vi "Build Caraya to PPL.vi"() -> ()   [LabVIEW 2020]
uses:
  <vilib>/AppBuilder/AB_API_Simple/Build (path).vi
  Caraya.lvlib
  <vilib>/AppBuilder/AB_API_Simple/NI_App_Builder_API.lvlib
panel:
  in  "Build Caraya PPL":bool
  in  "Destination Folder":path
  in  "Caraya PPL filename":string="Caraya"
  # "CARAYA PPL Builder\n\nFill in the destination folder and PPL filename."
  # ".lvlibp"
  # "Note: \nIt is recommended that you do not change the PPL filename."
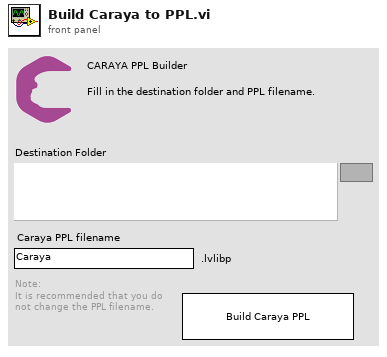
[diagram p1: front panel]
types:
  T1 = enum32{"invalid app kind", "Development System", "Run Time System", "Student Edition", "Embedded LabVIEW", "Evaluation", "Custom"}
  T2 = enum8{"Enabled", "Disabled", "Disabled and Grayed Out"}
  T3 = enum32{"Invalid", "Standard", "Closed", "Hidden", "Minimized", "Maximized"}
  T4 = cluster{"Core":cluster{"Current VI Reference":refnum<vi>, "Close Panel on Exit?":bool}, "PPL Filename":string, "Path":path, "Menu Launch AppRef":refnum<vi>, "Projects[]":refnum<vi>[]}
  T5 = cluster{"Current VI Reference":refnum<vi>, "Close Panel on Exit?":bool}
  T6 = typedef "Caraya.lvlib/Caraya Library Info.ctl" = cluster{"Version String":string, "Name":string, "Copyright":string, "License":string}
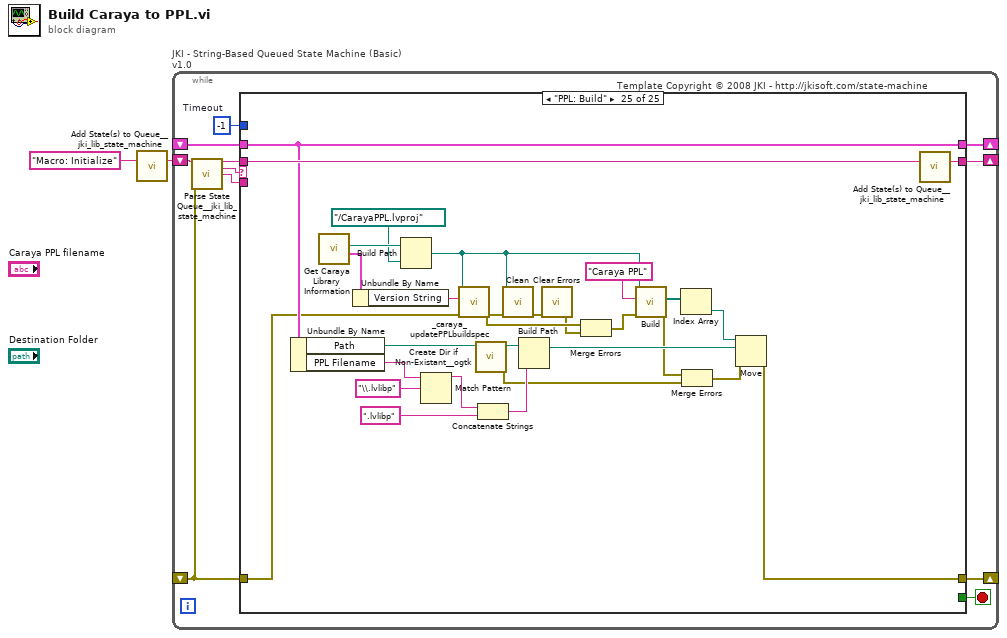
[diagram p0: block diagram]
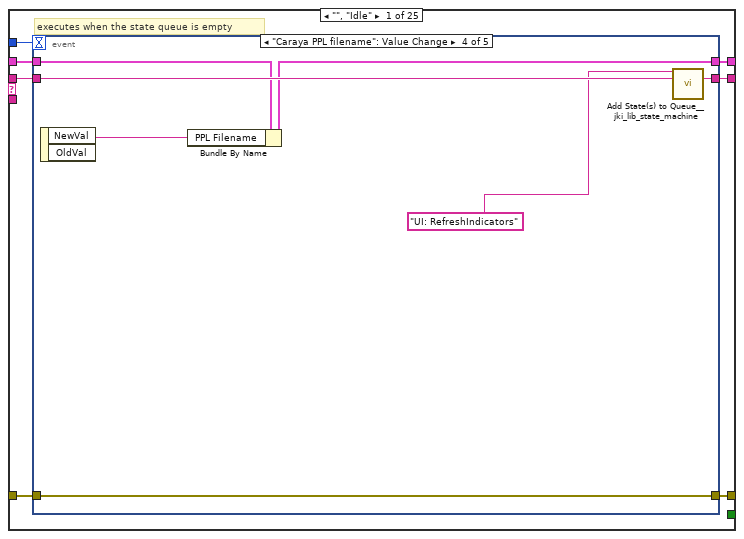
[diagram p2: hidden frame]
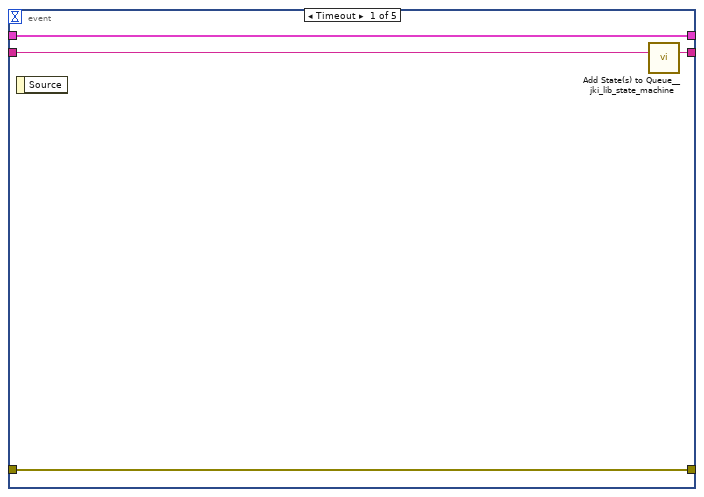
[diagram p3: hidden frame]
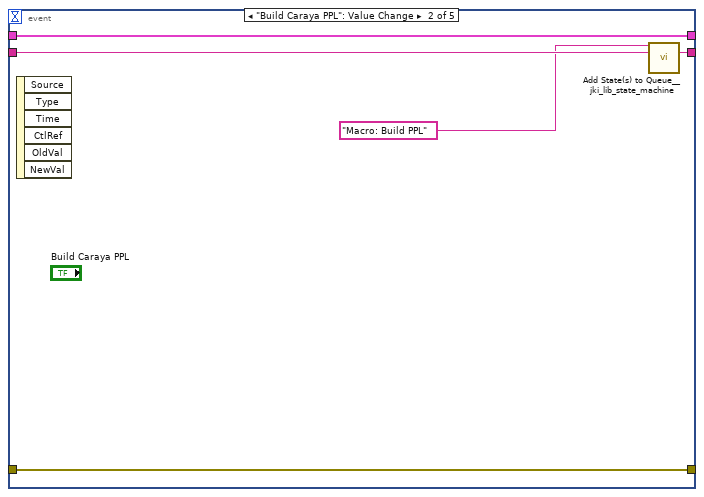
[diagram p4: hidden frame]
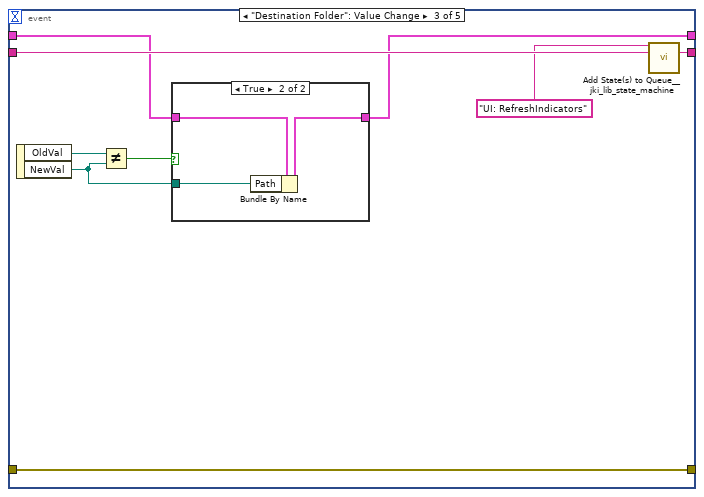
[diagram p5: hidden frame]
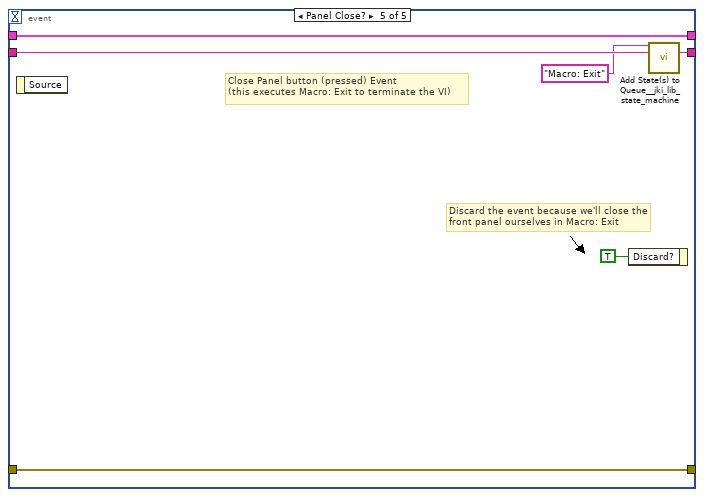
[diagram p7: hidden frame]
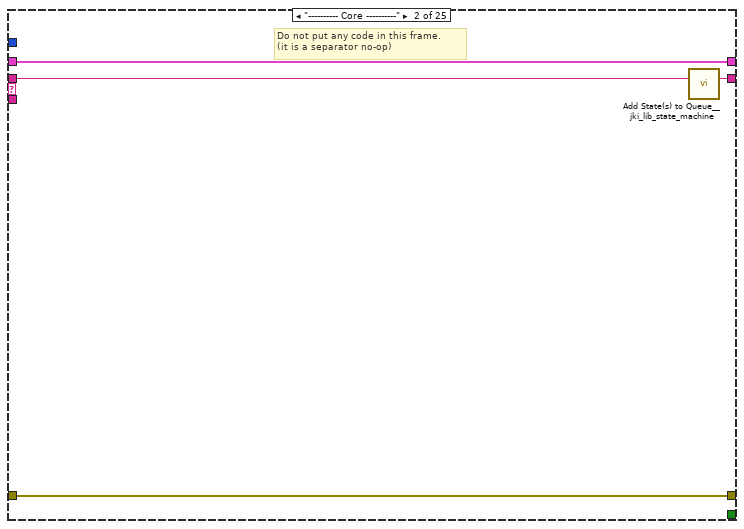
[diagram p8: hidden frame]
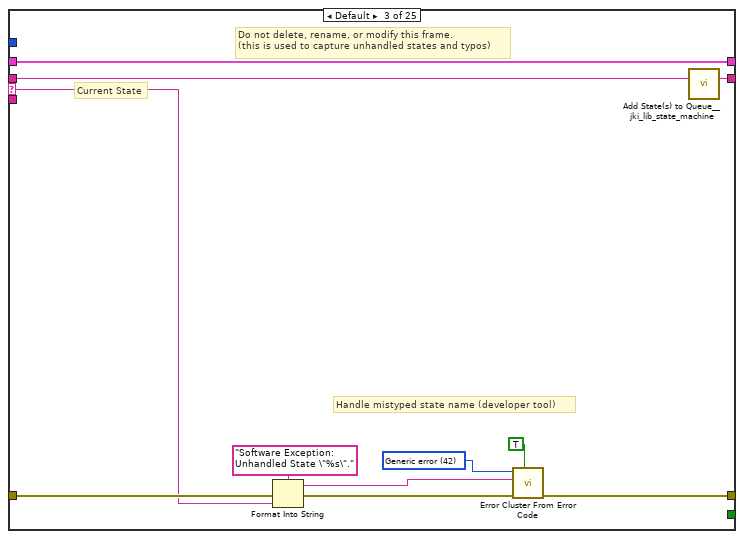
[diagram p9: hidden frame]
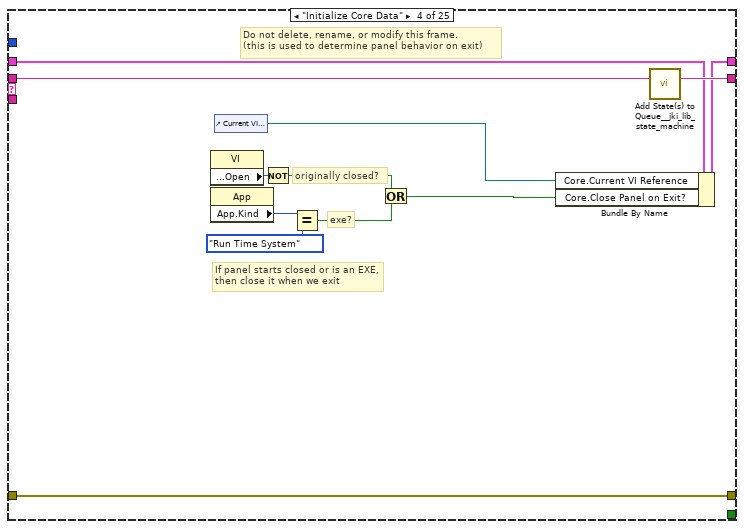
[diagram p10: hidden frame]
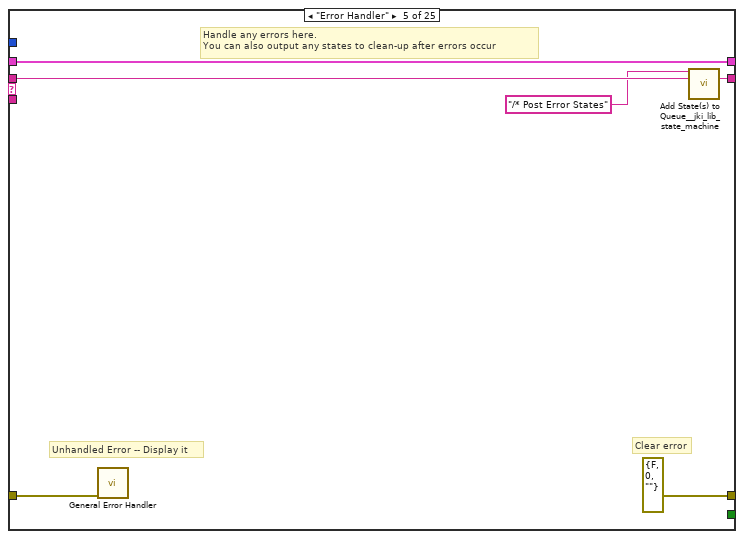
[diagram p11: hidden frame]
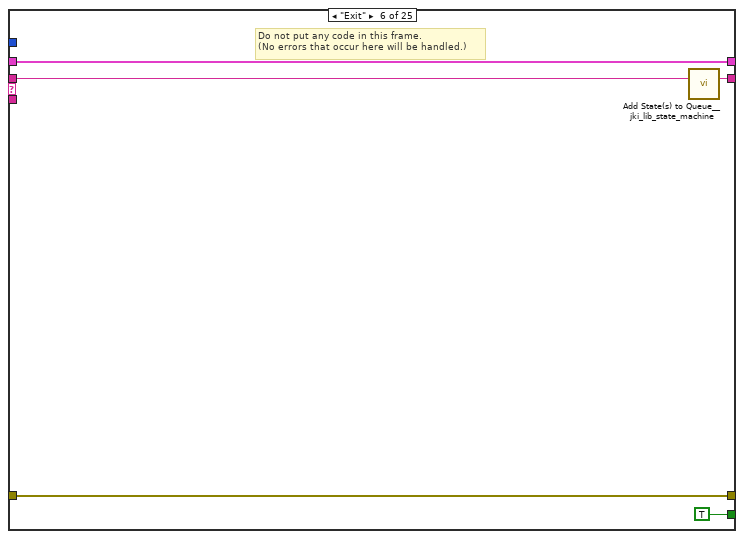
[diagram p12: hidden frame]
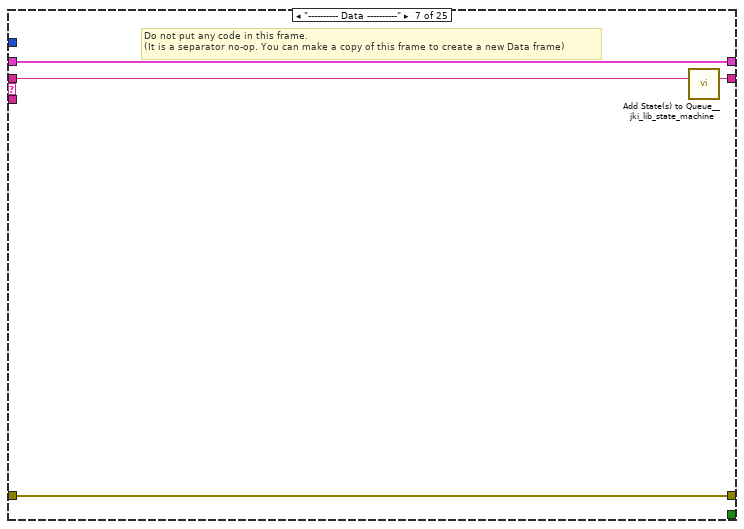
[diagram p13: hidden frame]
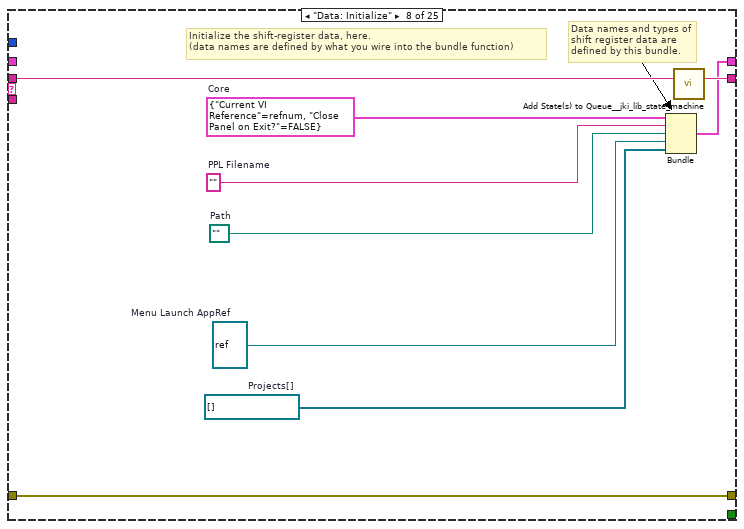
[diagram p14: hidden frame]
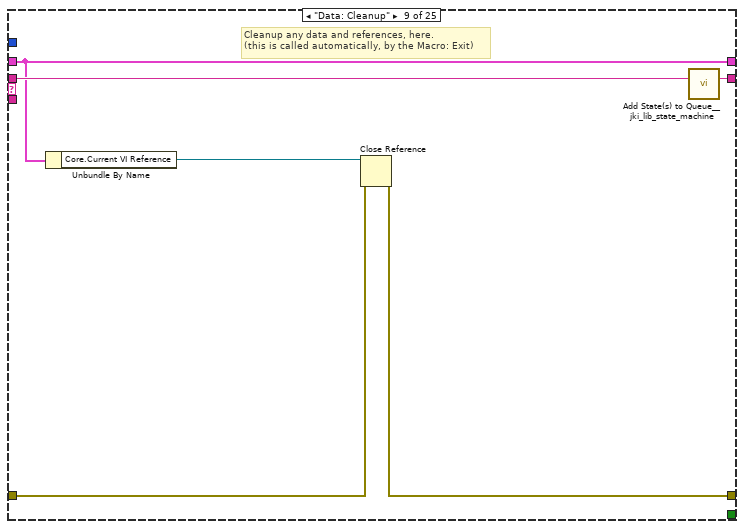
[diagram p15: hidden frame]
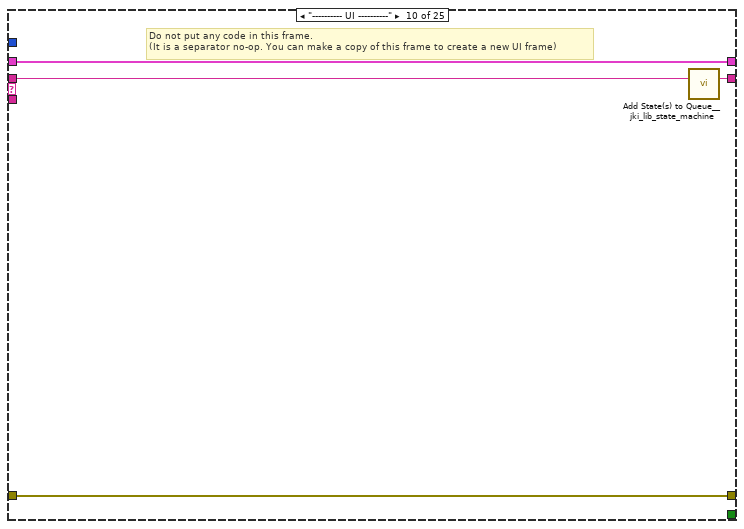
[diagram p16: hidden frame]
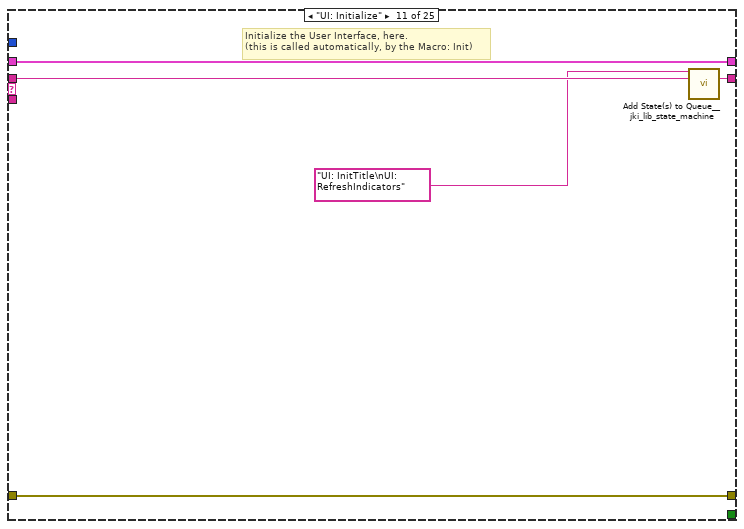
[diagram p17: hidden frame]
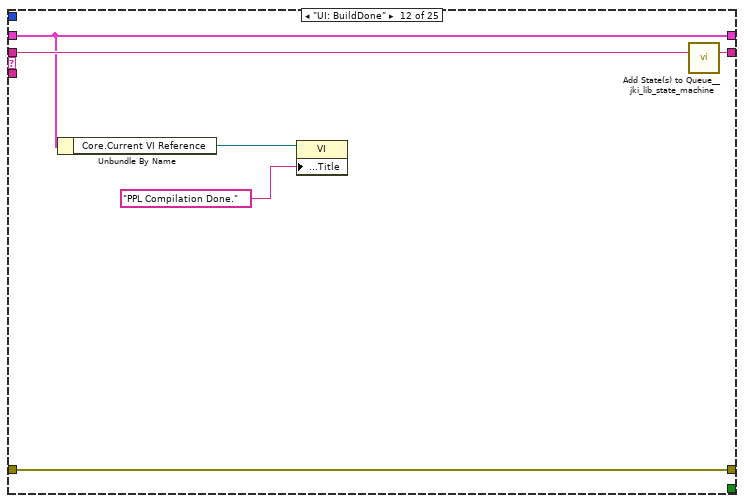
[diagram p18: hidden frame]
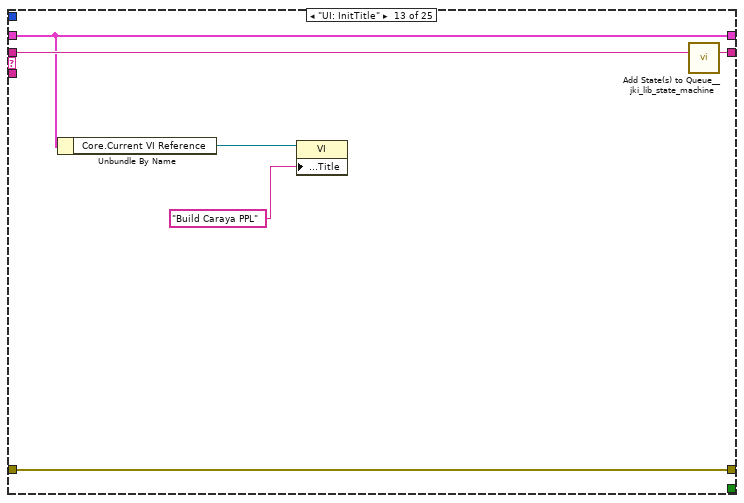
[diagram p19: hidden frame]
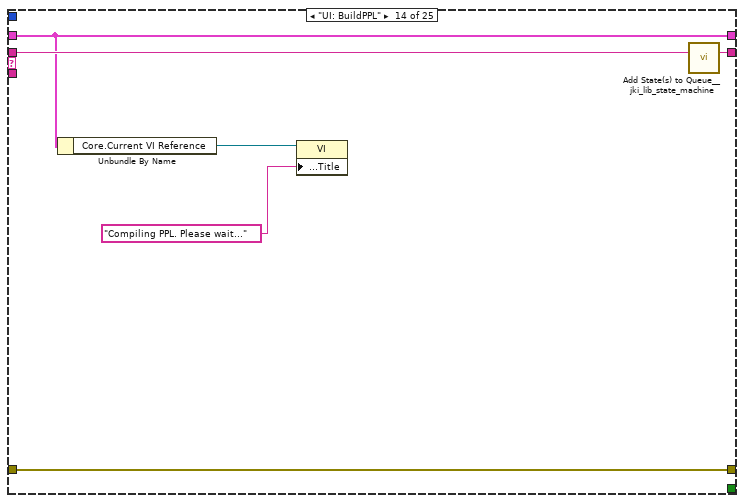
[diagram p20: hidden frame]
diagram:
  n1 = call <vilib>:"Add State(s) to Queue__jki_lib_state_machine.vi"("State(s) in (\"\")"="Macro: Initialize") -> ("States Out"=w2:string)  [unwired: 14 in]
  n2 = while "JKI - String-Based Queued State Machine (Basic) v1.0" {
    shift-right: [w6] -> _
    shift-left: _ -> [w5]
    shift-right: [w9] -> _
    shift-left: _ -> [w3]
    shift-right: [w8] -> _
    shift-left: w2 -> [w10]
    stop <- w7 stop-if-true
    w4 = -1  # Timeout
    # "Template Copyright © 2008 JKI - http://jkisoft.com/state-machine"
    n3 = call <vilib>:"Parse State Queue__jki_lib_state_machine.vi"("State Queue"=w10, "Error In (no error)"=w3) -> ("Remaining States"=w12:string, "Current State"=w13:string, "Arguments"=w11:string)  [unwired: 11 in]
    n4 = case shown="\"PPL: Build\"" w13 {
      selector: w13 -> [_ _ w60 _ _ _ _ _ _ _ _ _ _ _ _ _ _ _ _ _ _ _ _ _ _]
      tunnel: w12 -> [w20 w59 w64 w82 w88 w93 w97 w106 w112 w116 w121 w127 w133 w139 w152 w158 w169 w195 w200 w205 w212 w216 w222 w232 w262]
      tunnel: w11 -> [_ _ _ _ _ _ _ _ _ _ _ _ _ _ _ w153 w163 _ _ _ _ _ _ _ _]
      tunnel: w5 -> [w18 w56 w62 w73 w85 w91 w94 _ w107 w113 w118 w124 w130 w136 w140 w156 w165 w192 w197 w202 w209 w213 w218 w223 w260]
      tunnel: [w17 w57 w66 w79 errorcluster {"status"=FALSE, "code"=0, "source"=""} ("error out") w90 w95 w103 w108 w114 w119 w125 w131 w137 w150 w154 w166 w193 w198 w203 w210 w214 w220 w230 w241] -> w9
      tunnel: w3 -> [w16 w57 w65 w79 w84 w90 w95 w103 w109 w114 w119 w125 w131 w137 w150 w155 w167 w193 w198 w203 w210 w214 w220 w230 w247]
      tunnel: [w19 w58 w63 w81 w87 w92 w96 w105 w111 w115 w120 w126 w132 w138 w151 w157 w168 w194 w199 w204 w211 w215 w221 w231 w261] -> w8
      tunnel: [_ _ _ _ _ TRUE _ _ _ _ _ _ _ _ _ _ _ _ _ _ _ _ _ _ _] -> w7
      tunnel: [w15 w56 w62 w80 w85 w91 w94 w104 w107 w113 w118 w124 w130 w136 w140 w156 w165 w192 w197 w202 w209 w213 w217 w229 w260] -> w6
      tunnel: w4 -> [w14 _ _ _ _ _ _ _ _ _ _ _ _ _ _ _ _ _ _ _ _ _ _ _ _]
      frame "", "Idle" {
        # "executes when the state queue is empty"
        n5 = event shown="[3] \"Caraya PPL filename\": Value Change" {
          selector: _ -> [_ _ _ _ _]
          dyn-events: _ -> [_ _ _ _ _]
          timeout: w14 -> [_ _ _ _ _]
          tunnel: w20 -> [w24 w29 w38 w49 w55]
          tunnel: [w23 w28 w37 w48 w54] -> w19
          tunnel: w18 -> [w21 w26 w34 w46 w52]
          tunnel: [w22 w27 w36 w47 w53] -> w17
          tunnel: w16 -> [w22 w27 w36 w47 w53]
          tunnel: [w21 w26 w31 w45 w52] -> w15
          event Timeout {
            n6 = event-data() -> ()  [unwired: 1 in, 1 out]
            n7 = call <vilib>:"Add State(s) to Queue__jki_lib_state_machine.vi"("State(s) in (\"\")"=w24) -> ("States Out"=w23:string)  [unwired: 14 in]
          }
          event "Build Caraya PPL": Value Change {
            n8 = event-data() -> ()  [unwired: 1 in, 6 out]
            n9 = call <vilib>:"Add State(s) to Queue__jki_lib_state_machine.vi"("State(s) in Front (\"\")"="Macro: Build PPL", "State(s) in (\"\")"=w29) -> ("States Out"=w28:string)  [unwired: 13 in]
          }
          event "Destination Folder": Value Change {
            n10 = event-data() -> ("OldVal"=w35:path, "NewVal"=w32:path)  [unwired: 1 in]
            n11 = Not Equal?(x=w35, y=w32) -> (x != y?=w33:bool)
            n12 = case shown="True" w33 {
              tunnel: [w39 w42] -> w31
              tunnel: w34 -> [w39 w41]
              tunnel: w32 -> [_ w40]
              frame False {
              }
              frame True {
                n13 = Bundle By Name(cluster=w41, "Path"=w40) -> (w42:T4)
              }
            }
            n14 = call <vilib>:"Add State(s) to Queue__jki_lib_state_machine.vi"("State(s) in Front (\"\")"="UI: RefreshIndicators", "State(s) in (\"\")"=w38) -> ("States Out"=w37:string)  [unwired: 13 in]
          }
          event "Caraya PPL filename": Value Change {
            n15 = event-data() -> ("NewVal"=w44:string)  [unwired: 1 in, 1 out]
            n16 = Bundle By Name(cluster=w46, "PPL Filename"=w44) -> (w45:T4)
            n17 = call <vilib>:"Add State(s) to Queue__jki_lib_state_machine.vi"("State(s) in Front (\"\")"="UI: RefreshIndicators", "State(s) in (\"\")"=w49) -> ("States Out"=w48:string)  [unwired: 13 in]
          }
          event Panel Close? {
            # "Discard the event because we'll close the front panel ourselves in Macro: Exit"
            # "Close Panel button (pressed) Event\n(this executes Macro: Exit to terminate the VI)"
            n18 = event-data() -> ()  [unwired: 1 in, 1 out]
            n19 = event-data("Discard?"=TRUE) -> ()  [unwired: 1 in, 1 out]
            n20 = call <vilib>:"Add State(s) to Queue__jki_lib_state_machine.vi"("State(s) in Front (\"\")"="Macro: Exit", "State(s) in (\"\")"=w55) -> ("States Out"=w54:string)  [unwired: 13 in]
          }
        }
      }
      frame "---------- Core ----------" {
        # "Do not put any code in this frame.\n(it is a separator no-op)"
        n21 = call <vilib>:"Add State(s) to Queue__jki_lib_state_machine.vi"("State(s) in (\"\")"=w59) -> ("States Out"=w58:string)  [unwired: 14 in]
      }
      frame Default {
        w69 = 42 items=["No error", "Argument error", "Memory is full", "Out of zone", "End of file", "File already open", "Generic file I/O error", "File not found", "File permission error", "Disk is full", "Duplicate path", "Too many files open", "System feature not enabled", "Resource file not found", "Cannot add resource", "Resource not found", "Image not found", "Image memory error", "Pen does not exist", "Config type invalid", "Config token not found", "Config parse error", "Config memory error", "Bad external code format", "Bad external code offset", "External code not present", "Null window", "Destroy window error", "Null menu", "Print aborted", "Bad print record", "Print driver error", "Windows error during printing", "Memory error during printing", "Print dialog error", "Generic print error", "Invalid device refnum", "Device not found", "Device parameter error", "Device unit error", "Cannot open device", "Device call aborted", "Generic error", "Cancelled by user", "Object ID too low", "Object ID too high", "Object not in heap", "Unknown heap", "Unknown object (invalid DefProc)", "Unknown object (DefProc not in table)", "Message out of range", "Invalid (null) method", "Unknown message", "Manager call not supported", "Bad address", "Network operation in progress", "Network operation timed out", "Connection is busy", "Network attribute not supported", "Network error", "Address in use", "System out of memory", "Connection aborted", "Connection refused", "Not connected", "Already connected", "Connection closed", "Initialization error (interapplication manager)", "Bad occurrence", "Wait on unbound occurrence handler", "Occurrence queue overflow", "Datalog type conflict", "Unused", "Unrecognized type (interapplication manager)", "Memory corrupt", "Failed to make temporary DLL", "Old CIN version", "Drag socket not found", "Failed to load drop-object", "Failed to register OLE object", "Failed to release OLE object", "Format specifier type mismatch", "Unknown format specifier", "Too few format specifiers", "Too many format specifiers", "Scan failed", "Newer CIN version", "Error converting to variant", "Runtime menu error", "Password tampered", "Variant attribute not found", "Incompatible variant data type", "Event data is not available", "Event Store is not present", "Occurrence is not found", "Event Queue is not created", "Event info is not available", "Refnum passed is NULL", "Error retrieving Class GUID", "Error retrieving CoClass GUID", "Error retrieving TypeLib GUID.", "Bad built application magic bytes.", "Specific driver is different from the specific driver associated with the Logical Name.", "There is no session opened to the class driver.", "Max Error", "MAX - Error with config objects", "MAX - Error loading configuration", "MAX - Group not supported"]
        # "Current State"
        # "Do not delete, rename, or modify this frame.\n(this is used to capture unhandled states and typos)"
        # "Handle mistyped state name (developer tool)"
        n22 = Format Into String(format string="Software Exception: Unhandled State \"%s\"." ("message"), error in=w65, w60) -> (resulting string=w68:string, error out=w67:errorcluster)  [unwired: 1 in]
        n23 = call <vilib>:"Error Cluster From Error Code.vi"("show call chain? (False)"=TRUE, "error in (no error)"=w67, "error message (\"\")"=w68, "error code (0)"=w69) -> ("error out"=w66:errorcluster)  [unwired: 5 in]
        n24 = call <vilib>:"Add State(s) to Queue__jki_lib_state_machine.vi"("State(s) in (\"\")"=w64) -> ("States Out"=w63:string)  [unwired: 14 in]
      }
      frame "Initialize Core Data" {
        # "Do not delete, rename, or modify this frame.\n(this is used to determine panel behavior on exit)"
        # "originally closed?"
        # "exe?"
        # "If panel starts closed or is an EXE, then close it when we exit"
        n25 = property class="VI"() -> ("Front Panel.Open"=w78:bool)  [unwired: 2 in, 2 out]
        n26 = property class="App"() -> ("App.Kind"=w77:T1)  [unwired: 2 in, 2 out]
        n27 = control-ref of="Current VI Reference"() -> (w71:refnum<vi>)
        n28 = Not(x=w78) -> (.not. x?=w75:bool)
        n29 = Equal?(x=w77, y=T1."Run Time System" ("Application:Kind")) -> (x = y?=w74:bool)
        n30 = Or(x=w75, y=w74) -> (x .or. y?=w72:bool)
        n31 = Bundle By Name(cluster=w73, "Core.Current VI Reference"=w71, "Core.Close Panel on Exit?"=w72) -> (w80:T4)
        n32 = call <vilib>:"Add State(s) to Queue__jki_lib_state_machine.vi"("State(s) in (\"\")"=w82) -> ("States Out"=w81:string)  [unwired: 14 in]
      }
      frame "Error Handler" {
        # "Unhandled Error -- Display it"
        # "Handle any errors here.\nYou can also output any states to clean-up after errors occur"
        # "Clear error"
        n33 = call <vilib>:"General Error Handler.vi"("error in (no error)"=w84) -> ()  [unwired: 10 in, 5 out]
        n34 = call <vilib>:"Add State(s) to Queue__jki_lib_state_machine.vi"("State(s) in Front (\"\")"="/* Post Error States", "State(s) in (\"\")"=w88) -> ("States Out"=w87:string)  [unwired: 13 in]
      }
      frame "Exit" {
        # "Do not put any code in this frame.\n(No errors that occur here will be handled.)"
        n35 = call <vilib>:"Add State(s) to Queue__jki_lib_state_machine.vi"("State(s) in (\"\")"=w93) -> ("States Out"=w92:string)  [unwired: 14 in]
      }
      frame "---------- Data ----------" {
        # "Do not put any code in this frame.\n(It is a separator no-op. You can make a copy of this frame to create a new Data frame)"
        n36 = call <vilib>:"Add State(s) to Queue__jki_lib_state_machine.vi"("State(s) in (\"\")"=w97) -> ("States Out"=w96:string)  [unwired: 14 in]
      }
      frame "Data: Initialize" {
        w98 = refnum<vi>[] []  # Projects[]
        w99 = refnum<vi> refnum  # Menu Launch AppRef
        w100 = path ""  # Path
        w101 = T5 {"Current VI Reference"=refnum, "Close Panel on Exit?"=FALSE}  # Core
        w102 = ""  # PPL Filename
        # "Data names and types of shift register data are defined by this bundle."
        # "Initialize the shift-register data, here.\n(data names are defined by what you wire into the bundle function)"
        n37 = Bundle("Core"=w101, "PPL Filename"=w102, "Path"=w100, "Menu Launch AppRef"=w99, "Projects[]"=w98) -> (w104:T4)  [unwired: 1 in]
        n38 = call <vilib>:"Add State(s) to Queue__jki_lib_state_machine.vi"("State(s) in (\"\")"=w106) -> ("States Out"=w105:string)  [unwired: 14 in]
      }
      frame "Data: Cleanup" {
        # "Cleanup any data and references, here.\n(this is called automatically, by the Macro: Exit)"
        n39 = Unbundle By Name(w107) -> ("Core.Current VI Reference"=w110:refnum<vi>)
        n40 = Close Reference(reference=w110, error in (no error)=w109) -> (error out=w108:errorcluster)
        n41 = call <vilib>:"Add State(s) to Queue__jki_lib_state_machine.vi"("State(s) in (\"\")"=w112) -> ("States Out"=w111:string)  [unwired: 14 in]
      }
      frame "---------- UI ----------" {
        # "Do not put any code in this frame.\n(It is a separator no-op. You can make a copy of this frame to create a new UI frame)"
        n42 = call <vilib>:"Add State(s) to Queue__jki_lib_state_machine.vi"("State(s) in (\"\")"=w116) -> ("States Out"=w115:string)  [unwired: 14 in]
      }
      frame "UI: Initialize" {
        # "Initialize the User Interface, here.\n(this is called automatically, by the Macro: Init)"
        n43 = call <vilib>:"Add State(s) to Queue__jki_lib_state_machine.vi"("State(s) in Front (\"\")"="UI: InitTitle\nUI: RefreshIndicators" ("Text.Text"), "State(s) in (\"\")"=w121) -> ("States Out"=w120:string)  [unwired: 13 in]
      }
      frame "UI: BuildDone" {
        n44 = Unbundle By Name(w124) -> ("Core.Current VI Reference"=w123:refnum<vi>)
        n45 = property class="VI"(reference=w123, "Front Panel.Title"="PPL Compilation Done." ("Front Panel Window:Title")) -> ()  [unwired: 1 in, 2 out]
        n46 = call <vilib>:"Add State(s) to Queue__jki_lib_state_machine.vi"("State(s) in (\"\")"=w127) -> ("States Out"=w126:string)  [unwired: 14 in]
      }
      frame "UI: InitTitle" {
        n47 = Unbundle By Name(w130) -> ("Core.Current VI Reference"=w129:refnum<vi>)
        n48 = property class="VI"(reference=w129, "Front Panel.Title"="Build Caraya PPL" ("Front Panel Window:Title")) -> ()  [unwired: 1 in, 2 out]
        n49 = call <vilib>:"Add State(s) to Queue__jki_lib_state_machine.vi"("State(s) in (\"\")"=w133) -> ("States Out"=w132:string)  [unwired: 14 in]
      }
      frame "UI: BuildPPL" {
        n50 = Unbundle By Name(w136) -> ("Core.Current VI Reference"=w135:refnum<vi>)
        n51 = property class="VI"(reference=w135, "Front Panel.Title"="Compiling PPL. Please wait..." ("Front Panel Window:Title")) -> ()  [unwired: 1 in, 2 out]
        n52 = call <vilib>:"Add State(s) to Queue__jki_lib_state_machine.vi"("State(s) in (\"\")"=w139) -> ("States Out"=w138:string)  [unwired: 14 in]
      }
      frame "UI: RefreshIndicators" {
        n53 = Unbundle By Name(w140) -> ("PPL Filename"=w141:string, "Path"=w142:path)
        n54 = Empty String/Path?(string/path=w141) -> (empty?=w149:bool)
        n55 = Not A Number/Path/Refnum?(number/path/refnum=w142) -> (NaN/Path/Refnum?=w148:bool)
        n56 = Empty String/Path?(string/path=w142) -> (empty?=w147:bool)
        n57 = local write "Caraya PPL filename"(w141) -> ()
        n58 = local write "Destination Folder"(w142) -> ()
        n59 = Compound Arithmetic op=OR(w149, w148, w147) -> (w145:bool)
        n60 = Select(t=T2."Disabled and Grayed Out" ("Disabled"), s=w145, f=T2."Enabled" ("Disabled")) -> (s? t:f=w143:T2)
        n61 = property on="Build Caraya PPL" class="Bool"("DisabledEnum"=w143) -> ()  [unwired: 2 in, 2 out]
        n62 = call <vilib>:"Add State(s) to Queue__jki_lib_state_machine.vi"("State(s) in (\"\")"=w152) -> ("States Out"=w151:string)  [unwired: 14 in]
      }
      frame "UI: Cursor Set" {
        # "Argument"
        # "Set and Unset Cursor Busy.\n(Usage: \"UI: Cursor Set >> Busy|Idle\")"
        n63 = case shown="\"Idle\", Default" w153 {
          tunnel: w155 -> [w160 w162]
          tunnel: [w159 w161] -> w154
          frame "Idle", Default {
            n64 = call <vilib>:"Unset Busy.vi"("error in (no error)"=w160) -> ("error out"=w159:errorcluster)  [unwired: 10 in]
          }
          frame "Busy" {
            n65 = call <vilib>:"Set Busy.vi"("error in (no error)"=w162) -> ("error out"=w161:errorcluster)  [unwired: 9 in, 1 out]
          }
        }
        n66 = call <vilib>:"Add State(s) to Queue__jki_lib_state_machine.vi"("State(s) in (\"\")"=w158) -> ("States Out"=w157:string)  [unwired: 14 in]
      }
      frame "UI: Front Panel State" {
        # "Argument"
        # "Set Front Panel Open or Closed\n(Usage: \"UI: Front Panel State >> Open|Close\")"
        n67 = Unbundle By Name(w165) -> ("Core.Current VI Reference"=w164:refnum<vi>)
        n68 = case shown="\"Open\", Default" w163 {
          tunnel: w167 -> [w173 w186]
          tunnel: [w175 w187] -> w166
          tunnel: w164 -> [w174 w184]
          frame "Open", Default {
            n69 = property class="VI"(reference=w174, error in=w173) -> (reference out=w171:refnum<vi>, error out=w172:errorcluster, "Front Panel.Open"=w170:bool)
            n70 = case shown="False" w170 {
              tunnel: [w178 w181] -> w175
              tunnel: w172 -> [w177 w181]
              tunnel: w171 -> [w176 _]
              frame False {
                n71 = invoke class="VI" method="FP.Open"(reference=w176, error in=w177, "Activate"=TRUE, "State"=T3."Standard") -> (error out=w178:errorcluster)  [unwired: 1 in, 4 out]
              }
              frame True {
              }
            }
          }
          frame "Close" {
            n72 = property class="VI"(reference=w184, error in=w186) -> (reference out=w183:refnum<vi>, error out=w185:errorcluster, "Front Panel.Open"=w182:bool)
            n73 = case shown="True" w182 {
              tunnel: [w188 w191] -> w187
              tunnel: w185 -> [w188 w190]
              tunnel: w183 -> [_ w189]
              frame False {
              }
              frame True {
                n74 = invoke class="VI" method="FP.Close"(reference=w189, error in=w190) -> (error out=w191:errorcluster)  [unwired: 1 in, 2 out]
              }
            }
          }
        }
        n75 = call <vilib>:"Add State(s) to Queue__jki_lib_state_machine.vi"("State(s) in (\"\")"=w169) -> ("States Out"=w168:string)  [unwired: 14 in]
      }
      frame "---------- Macro ----------" {
        # "Do not put any code in this frame.\n(It is a separator no-op. You can make a copy of this frame to create a new Macro frame)"
        n76 = call <vilib>:"Add State(s) to Queue__jki_lib_state_machine.vi"("State(s) in (\"\")"=w195) -> ("States Out"=w194:string)  [unwired: 14 in]
      }
      frame "Macro: Initialize" {
        w196 = "Data: Initialize\nInitialize Core Data\nPPL: Initialize Filename\nPPL: Initialize Path\nUI: Initialize\nUI: Front Panel State >> Open"  # Data: Initialize Initialize Core Data PPL: Initialize Filename PPL: Initialize Path UI: Initialize UI: Front Panel State >> Open
        # "Initialization Macro\n(This is called once, when the VI starts)"
        n77 = call <vilib>:"Add State(s) to Queue__jki_lib_state_machine.vi"("State(s) in Front (\"\")"=w196, "State(s) in (\"\")"=w200) -> ("States Out"=w199:string)  [unwired: 13 in]
      }
      frame "Macro: Build PPL" {
        n78 = call <vilib>:"Add State(s) to Queue__jki_lib_state_machine.vi"("State(s) in Front (\"\")"="UI: BuildPPL\nPPL: Build\nUI: BuildDone", "State(s) in (\"\")"=w205) -> ("States Out"=w204:string)  [unwired: 13 in]
      }
      frame "Macro: Exit" {
        # "Exit Macro\n(This is called once, when the VI exits)"
        n79 = call <vilib>:"Add State(s) to Queue__jki_lib_state_machine.vi"("State(s) in Front (\"\")"="UI: Front Panel State >> Close", "State(s) at Back (\"\")"="Data: Cleanup\nExit") -> ("States Out"=w207:string)  [unwired: 13 in]
        n80 = call <vilib>:"Add State(s) to Queue__jki_lib_state_machine.vi"("State(s) in Front (\"\")"=w207, "State(s) in (\"\")"=w212) -> ("States Out"=w211:string)  [unwired: 13 in]
      }
      frame "---------- PPL ----------" {
        n81 = call <vilib>:"Add State(s) to Queue__jki_lib_state_machine.vi"("State(s) in (\"\")"=w216) -> ("States Out"=w215:string)  [unwired: 14 in]
      }
      frame "PPL: Initialize Filename" {
        n82 = Unbundle By Name(w218) -> ()  [unwired: 1 out]
        n83 = Bundle By Name(cluster=w218, "PPL Filename"="Caraya") -> (w217:T4)
        n84 = call <vilib>:"Add State(s) to Queue__jki_lib_state_machine.vi"("State(s) in (\"\")"=w222) -> ("States Out"=w221:string)  [unwired: 14 in]
      }
      frame "PPL: Initialize Path" {
        n85 = property on="Destination Folder" class="Path"() -> ("Value"=w225:path)  [unwired: 2 in, 2 out]
        n86 = Not A Number/Path/Refnum?(number/path/refnum=w225) -> (NaN/Path/Refnum?=w224:bool)
        n87 = Empty String/Path?(string/path=w225) -> (empty?=w227:bool)
        n88 = Or(x=w224, y=w227) -> (x .or. y?=w226:bool)
        n89 = case shown="True" w226 {
          tunnel: w225 -> [w233 _]
          tunnel: [w233 w234] -> w228
          frame False {
          }
          frame True {
            n90 = call <vilib>:"Application Directory.vi"() -> ("Application Directory"=w234:path)
          }
        }
        n91 = Bundle By Name(cluster=w223, "Path"=w228) -> (w229:T4)
        n92 = call <vilib>:"Add State(s) to Queue__jki_lib_state_machine.vi"("State(s) in (\"\")"=w232) -> ("States Out"=w231:string)  [unwired: 14 in]
      }
      frame "PPL: Build" {
        n93 = Unbundle By Name(w260) -> ("Path"=w246:path, "PPL Filename"=w239:string)
        n94 = call "Get Caraya Library Information.vi"() -> ("Library Info"=w256:T6, "Caraya Library Path"=w259:path)  [unwired: 9 in, 1 out]
        n95 = Unbundle By Name(w256) -> ("Version String"=w255:string)
        n96 = Build Path(base path=w259, name or relative path=path "../CarayaPPL.lvproj" ("Caraya Library Path")) -> (appended path=w254:path)
        n97 = Match Pattern(string=w239, regular expression="\\.lvlibp") -> (before substring=w251:string)  [unwired: 1 in, 3 out]
        n98 = call "_caraya_updatePPLbuildspec.vi"("error in (no error)"=w247, "Version"=w255, "Project Path"=w254) -> ("error out"=w237:errorcluster)  [unwired: 8 in]
        n99 = call <userlib>:"Create Dir if Non-Existant__ogtk.vi"("Directory Path"=w246) -> ("error out"=w244:errorcluster, "dup Directory Path"=w245:path)  [unwired: 8 in, 1 out]
        n100 = Concatenate Strings(w251, ".lvlibp" ("regular expression")) -> (w249:string)
        n101 = call <vilib>:"Clean.vi"("error in (no error)"=w237, "Path to project"=w254) -> ("error out"=w238:errorcluster)  [unwired: 9 in]
        n102 = Build Path(base path=w245, name or relative path=w249) -> (appended path=w248:path)
        n103 = call <vilib>:"Clear Errors.vi"("error in (no error)"=w238) -> ("error out"=w236:errorcluster)  [unwired: 5 in, 1 out]
        n104 = Merge Errors(w237, w236) -> (w235:errorcluster)
        n105 = call-poly <vilib>:"Build.vi"("error in (no error)"=w235, "Name of build specification (if empty: build all)"="Caraya PPL", "Path to project"=w254) -> ("error out"=w243:errorcluster, "Generated files"=w253:path[])  [unwired: 7 in]
        n106 = Index Array(array=w253) -> (element=w240:path)  [unwired: 1 in]
        n107 = Merge Errors(w243, w244) -> (w242:errorcluster)
        n108 = Move(source path=w240, error in=w242, 10:w248) -> (error out=w241:errorcluster)  [unwired: 2 in, 2 out]
        n109 = call <vilib>:"Add State(s) to Queue__jki_lib_state_machine.vi"("State(s) in (\"\")"=w262) -> ("States Out"=w261:string)  [unwired: 14 in]
      }
    }
  }
